vi "Test WS.vi"(7 "LabVIEW Web Service Request":refnum<class "Web Request.lvclass">, 11 "value":string) -> (3 "x = y?":bool)   [LabVIEW 2014]
uses:
  <vilib>/wsapi/Web Request.lvclass
  <vilib>/wsapi/class/subVIs/Write Single Session Variable.vi
panel:
  out "value 2":string
  out "session ID cookie":string
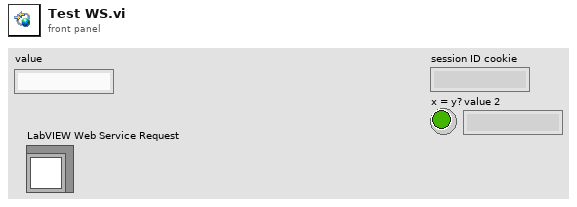
[diagram p1: front panel]
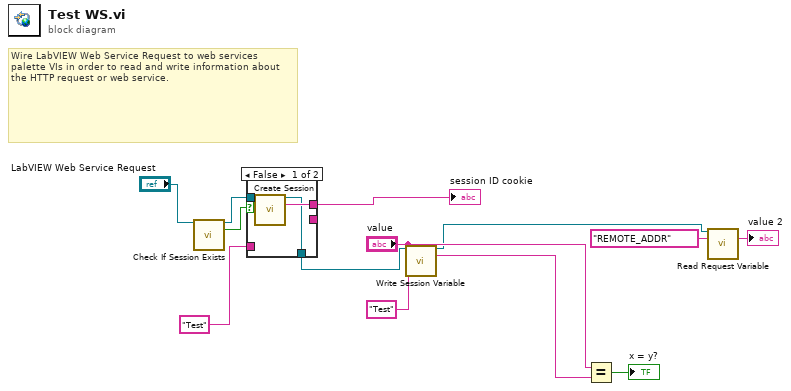
[diagram p0: block diagram]
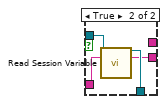
[diagram p2: hidden frame]
diagram:
  # "Wire LabVIEW Web Service Request to web services palette VIs in order to read and write information about the HTTP request or web service."
  n1 = call <vilib>:"Check If Session Exists.vi"("LabVIEW Web Service Request"="LabVIEW Web Service Request") -> ("LabVIEW Web Service Request out"=w10:refnum<class "Web Request.lvclass">, "session exists?"=w9:bool)  [unwired: 12 in, 1 out]
  n2 = case shown="False" w9 {
    tunnel: [w16 _] -> w13
    tunnel: w10 -> [w15 w20]
    tunnel: [w14 w19] -> w8
    tunnel: "Test" ("key") -> [_ w18]
    tunnel: [_ w17] -> _
    frame False {
      n3 = call <vilib>:"Create Session.vi"("LabVIEW Web Service Request"=w15) -> ("LabVIEW Web Service Request out"=w14:refnum<class "Web Request.lvclass">, "session ID cookie"=w16:string)  [unwired: 12 in, 1 out]
    }
    frame True {
      n4 = call <vilib>:"Read Session Variable.vi"("LabVIEW Web Service Request"=w20, "key"=w18) -> ("LabVIEW Web Service Request out"=w19:refnum<class "Web Request.lvclass">, "value"=w17:string)  [unwired: 11 in, 1 out]
    }
  }
  "session ID cookie" <- w13
  n5 = call-poly <vilib>:"Write Session Variable.vi"("LabVIEW Web Service Request"=w8, "key"="Test", "value"="value") -> ("LabVIEW Web Service Request out"=w2:refnum<class "Web Request.lvclass">, "previous value"=w5:string)  [unwired: 9 in, 2 out]
  n6 = Equal?(x="value", y=w5) -> (x = y?=→"x = y?":bool)
  n7 = call <vilib>:"Read Request Variable.vi"("LabVIEW Web Service Request"=w2, "variable name"="REMOTE_ADDR") -> ("value"=→"value 2":string)  [unwired: 11 in, 2 out]
